vi "Straightened Arcade.vi"(11 "Metrics In":T2={"Timestamp"=0, "Drive State"=enum."Initialize", "Throttle"=-0.0, "Turn"=0.0, "Heading"=0.0, "Absolute Heading"=0.0, "Left Velocity"=0.0, "Left Encoder"=0.0, "Right Velocity"=0.0, "Right Encoder"=0.0, "Left Power"=7.353305345843318, "Right Power"=-7.353305345843318, "Last Shift"=0, "Shift Started"=0, "Duration"=0, "Copilot State"=enum."None", "Collect Power"=0.0, "Flywheel Power Left"=0.0, "Flywheel Power Right"=0.0}) -> (3 "Metrics Out":T2={"Timestamp"=0, "Drive State"=enum."Initialize", "Throttle"=-0.0, "Turn"=7.353785345866117, "Heading"=0.0, "Absolute Heading"=0.0, "Left Velocity"=0.0, "Left Encoder"=0.0, "Right Velocity"=0.0, "Right Encoder"=0.0, "Left Power"=7.353785345866117, "Right Power"=-7.353785345866117, "Last Shift"=0, "Shift Started"=0, "Duration"=0, "Copilot State"=enum."None", "Collect Power"=0.0, "Flywheel Power Left"=0.0, "Flywheel Power Right"=0.0})   [LabVIEW 2015]
uses:
  Drive Metrics.ctl
  Drive States.ctl
  Copilot States.ctl
  Support/LightningPID Settings.ctl
  Support/Global Objects.vi
panel:
  in  "PID Settings":T1={"iMax"=0.1, "iMin"=-0.1, "iGain"=0.0, "pGain"=0.0, "dGain"=0.0, "MaxOutput"=1.0, "MinOutput"=-1.0, "AutoReset"=FALSE, "Tolerance"=2.0, "dSmoothing"=0.0}
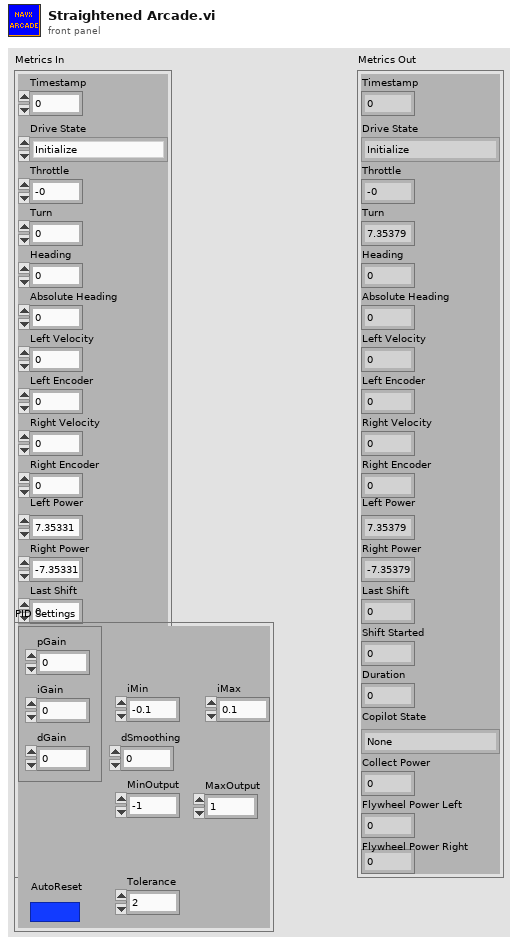
[diagram p1: front panel]
types:
  T1 = typedef "LightningPID Settings.ctl" = cluster{"iMax":dbl, "iMin":dbl, "iGain":dbl, "pGain":dbl, "dGain":dbl, "MaxOutput":dbl, "MinOutput":dbl, "AutoReset":bool, "Tolerance":dbl, "dSmoothing":dbl}
  T2 = typedef "Drive Metrics.ctl" = cluster{"Timestamp":u32, "Drive State":T3, "Throttle":dbl, "Turn":dbl, "Heading":dbl, "Absolute Heading":dbl, "Left Velocity":dbl, "Left Encoder":dbl, "Right Velocity":dbl, "Right Encoder":dbl, "Left Power":dbl, "Right Power":dbl, "Last Shift":u32, "Shift Started":u32, "Duration":i64, "Copilot State":T4, "Collect Power":dbl, "Flywheel Power Left":dbl, "Flywheel Power Right":dbl}
  T3 = typedef "Drive States.ctl" = enum16{"Initialize", "Low Gear", "Up Shift Begin", "Up Shifting", "Up Shift Delay", "High Gear", "Down Shift Begin", "Down Shifting", "Down Shift Delay"}
  T4 = typedef "Copilot States.ctl" = enum16{"None", "Collect", "Eject"}
  T5 = typedef "Configuration.ctl" = cluster{"Throttle Dead Zone":dbl, "Throttle Ramp Rate":dbl, "Turn Dead Zone":dbl, "Auton":cluster{"Motion Plan P":dbl, "Motion Plan I":dbl, "Motion Plan D":dbl}, "Auto Upshift Enabled":bool, "Upshift Min Throttle":dbl, "Upshift Min Velocity":dbl, "Min time before upshift":dbl, "Shift Throttle Detent":u32, "Min time before downshift":dbl, "Turn PID":cluster{"Motion Plan P":dbl, "Motion Plan I":dbl, "Motion Plan D":dbl}, "Auto Coast Downshift":bool, "Downshift Coast Max Vel":dbl, "Downshift Coast Throttle Epsilon":dbl}
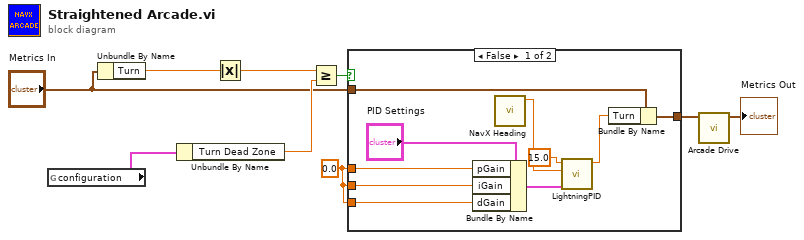
[diagram p0: block diagram]
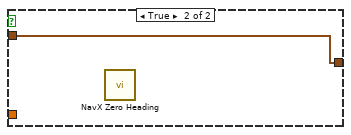
[diagram p2: hidden frame]
diagram:
  w1 = 0.0 ("Motion Plan P")
  n1 = global read "Global Objects.vi" "configuration"() -> (w8:T5)
  n2 = Unbundle By Name("Metrics In") -> ("Turn"=w7:dbl)
  n3 = Unbundle By Name(w8) -> ("Turn Dead Zone"=w6:dbl)
  n4 = Absolute Value(x=w7) -> (abs(x)=w2:dbl)
  n5 = Greater Or Equal?(x=w2, y=w6) -> (x >= y?=w5:bool)
  n6 = case shown="False" w5 {
    tunnel: [w18 w20] -> w4
    tunnel: "Metrics In" -> [w19 w20]
    tunnel: w1 -> [w17 _]
    tunnel: w1 -> [w16 _]
    tunnel: w1 -> [w15 _]
    frame False {
      n7 = Bundle By Name(cluster="PID Settings", "pGain"=w17, "iGain"=w16, "dGain"=w15) -> (w10:T1)
      n8 = call "NavX Heading.vi"() -> ("Heading"=w12:dbl)  [unwired: 9 in, 2 out]
      n9 = call "LightningPID.vi"("PID Settings"=w10, "Position"=w12, "Set Point"=15.0) -> ("Output"=w13:dbl)  [unwired: 8 in]
      n10 = Bundle By Name(cluster=w19, "Turn"=w13) -> (w18:T2)
    }
    frame True {
      n11 = call "NavX Zero Heading.vi"() -> ()  [unwired: 11 in, 1 out]
    }
  }
  n12 = call "Arcade Drive.vi"("Metrics In"=w4) -> ("Metrics Out"=→"Metrics Out":T2)  [unwired: 6 in]
